vi "OAT Polar Plot Cursor on Picture.vi"(6 "cursor attributes":T2={"layout color"=852223, "active color"=16740820, "precision"=2, "BG transparent? (T)"=FALSE, "radius"=2}, 7 "polar settings":T4={"polar attributes"={"maximum"=2.0, "minimum"=0.0, "clip to min"=FALSE, "log"=FALSE, "grid color"=3381657, "plot color"=16711680, "fmt and prec"={"format"=enum."Decimal", "precision"=2}, "visible section"=4}, "desired font"=enum."Application Font", "user-specified font"={"Font Name:"="", "Size"=0, "Strikeout?"=FALSE, "Italic?"=FALSE, "Underline?"=FALSE, "Outline?"=FALSE, "Shadow?"=FALSE, "Bold?"=FALSE}} {"polar attributes"."minimum" format="%.2f"; "polar attributes"."maximum" format="%.2f"}, 8 "avoid overlap? (Y)":bool=TRUE, 9 "grid measurements in":T1 {"end angle" format="%.2f"; "start angle" format="%.2f"; "scale factors"."b" format="%.2f"; "scale factors"."a" format="%.2f"}, 10 "Cursor List":T3(array[cluster]) {"Location"."Y" format="%.2f"; "Location"."X" format="%.2f"}, 11 "picture":picture) -> (1 "grid measurements out":T1 {"end angle" format="%.2f"; "start angle" format="%.2f"; "scale factors"."b" format="%.2f"; "scale factors"."a" format="%.2f"}, 3 "new picture":picture)   [LabVIEW 2017]
uses:
  <vilib>/addons/Sound and Vibration/Order Analysis/Backward Compatibility/SubVIs/OAT Polar Cursor Attributes.ctl
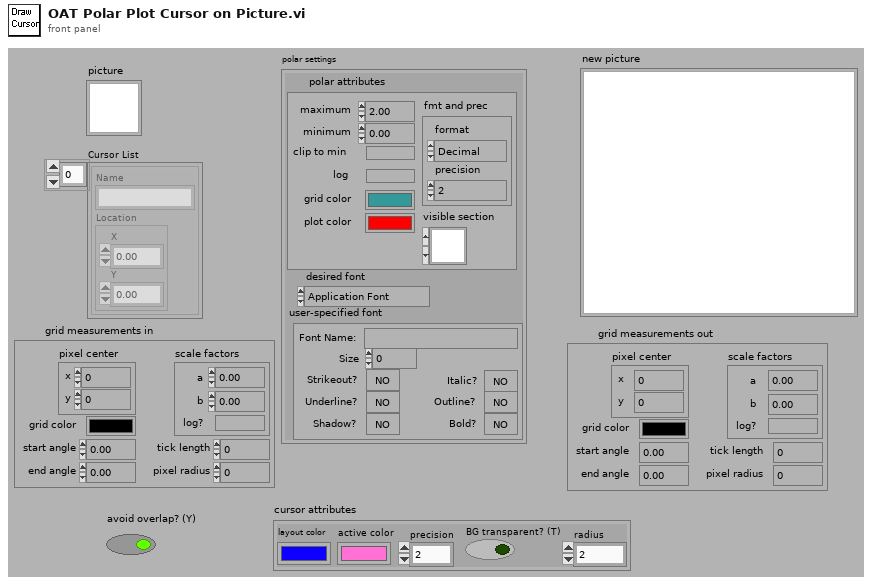
[diagram p1: front panel]
types:
  T1 = cluster{"pixel center":cluster{"x":i16, "y":i16}, "scale factors":cluster{"a":dbl, "b":dbl, "log?":bool}, "grid color":u32, "start angle":dbl, "end angle":dbl, "tick length":i16, "pixel radius":i32}
  T2 = typedef "OAT Polar Cursor Attributes.ctl" = cluster{"layout color":u32, "active color":u32, "precision":i16, "BG transparent? (T)":bool, "radius":i16}
  T3 = cluster{"Name":string, "Location":cluster{"X":dbl, "Y":dbl}}[]
  T4 = cluster{"polar attributes":cluster{"maximum":dbl, "minimum":dbl, "clip to min":bool, "log":bool, "grid color":u32, "plot color":u32, "fmt and prec":cluster{"format":enum8{"Decimal", "Scientific", "Engineering", "Binary", "Octal", "Hex"}, "precision":u8}, "visible section":u16}, "desired font":enum16{"User-specified Font", "Application Font", "System Font", "Dialog Font"}, "user-specified font":cluster{"Font Name:":string, "Size":i16, "Strikeout?":bool, "Italic?":bool, "Underline?":bool, "Outline?":bool, "Shadow?":bool, "Bold?":bool}}
  T5 = cluster{"left":i16, "top":i16, "right":i16, "bottom":i16}[]
  T6 = cluster{"maximum":dbl, "minimum":dbl, "clip to min":bool, "log":bool, "grid color":u32, "plot color":u32, "fmt and prec":cluster{"format":enum8{"Decimal", "Scientific", "Engineering", "Binary", "Octal", "Hex"}, "precision":u8}, "visible section":u16}
  T7 = enum16{"User-specified Font", "Application Font", "System Font", "Dialog Font"}
  T8 = cluster{"Font Name:":string, "Size":i16, "Strikeout?":bool, "Italic?":bool, "Underline?":bool, "Outline?":bool, "Shadow?":bool, "Bold?":bool}
  T9 = cluster{"left":i16, "top":i16, "right":i16, "bottom":i16}
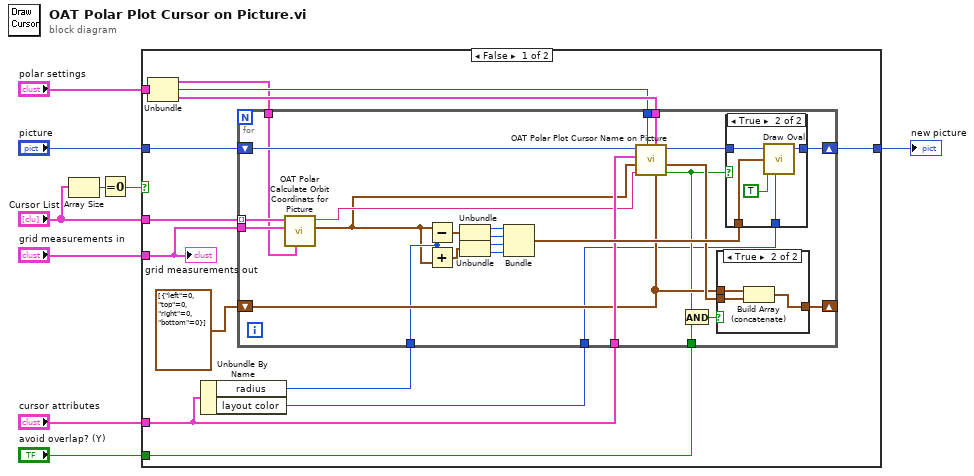
[diagram p0: block diagram]
diagram:
  n1 = Array Size(array="Cursor List") -> (size(s)=w2:i32)
  n2 = Equal To 0?(x=w2) -> (x = 0?=w1:bool)
  n3 = case shown="False" w1 {
    tunnel: "picture" -> [w22 w59]
    tunnel: [w20 w59] -> w8
    tunnel: "avoid overlap? (Y)" -> [w19 _]
    tunnel: "cursor attributes" -> [w17 _]
    tunnel: "polar settings" -> [w15 _]
    tunnel: "grid measurements in" -> [w11 _]
    tunnel: "Cursor List" -> [w10 _]
    frame False {
      n4 = Unbundle(w15) -> ("polar attributes"=w12:T6, "desired font"=w13:T7, "user-specified font"=w14:T8)
      n5 = Unbundle By Name(w17) -> ("radius"=w16:i16, "layout color"=w21:u32)
      n6 = for {
        tunnel: w10 -> [w25] mode=indexing
        shift-right: [w37] -> w20
        shift-left: w22 -> [w36]
        tunnel: w21 -> [w35]
        tunnel: w16 -> [w34]
        tunnel: w13 -> [w47]
        tunnel: w14 -> [w46]
        tunnel: w17 -> [w45]
        shift-right: [w41] -> _
        shift-left: T5 [{"left"=0, "top"=0, "right"=0, "bottom"=0}] -> [w40]
        tunnel: w19 -> [w43]
        tunnel: w11 -> [w24]
        tunnel: w12 -> [w23]
        n7 = call <vilib>:"OAT Polar Calculate Orbit Coordinats for Picture.vi"("polar attributes"=w23, "grid measurements"=w24, 11:w25) -> ("position"=w26:cluster{"x":i16, "y":i16}, "Name"=w27:string)  [unwired: 7 in]
        n8 = Subtract(x=w26, y=w34) -> (x-y=w32:cluster{"x":i16, "y":i16})
        n9 = Add(x=w34, y=w26) -> (x+y=w33:cluster{"x":i16, "y":i16})
        n10 = Unbundle(w32) -> ("x"=w31:i16, "y"=w30:i16)
        n11 = Unbundle(w33) -> ("x"=w29:i16, "y"=w28:i16)
        n12 = Bundle("x"=w31, "y"=w30, "x"=w29, "y"=w28) -> (w48:cluster{"x":i16, "y":i16, "x":i16, "y":i16})  [unwired: 1 in]
        n13 = call <vilib>:"OAT Polar Plot Cursor Name on Picture.vi"("avoid rect"=w40, "[user-specified font]"=w46, "desired font(Application)"=w47, "name"=w27, "cursor position"=w26, "cursor attributes"=w45, "picture"=w36) -> ("text plotted"=w39:bool, "text rect"=w42:T9, "new picture"=w38:picture)  [unwired: 2 in]
        n14 = And(x=w39, y=w43) -> (x .and. y?=w44:bool)
        n15 = case shown="True" w44 {
          tunnel: w42 -> [_ w58]
          tunnel: [w55 w57] -> w41
          tunnel: w40 -> [w55 w56]
          frame False {
          }
          frame True {
            n16 = Build Array (concatenate)(w56, w58) -> (w57:T5)
          }
        }
        n17 = case shown="True" w39 {
          tunnel: w38 -> [w49 w54]
          tunnel: [w49 w53] -> w37
          tunnel: w48 -> [_ w52]
          tunnel: w35 -> [_ w51]
          frame False {
          }
          frame True {
            n18 = call <vilib>:"Draw Oval.vi"("picture"=w54, "rect"=w52, "fill?(F)"=TRUE, "color(black)"=w51) -> ("new picture"=w53:picture)  [unwired: 5 in]
          }
        }
      }
      "grid measurements out" <- w11
    }
    frame True {
    }
  }
  "new picture" <- w8
